vi "Bias Shift.vi"(8 "y":dbl, 9 "x":dbl, 11 "Dx, Dy":cluster{"Dx":sgl, "Dy":sgl}={"Dx"=1e-10, "Dy"=1e-10}) -> (2 "Y (m)":sgl format="%.3p", 3 "X (m)":sgl format="%.3p")   [LabVIEW 2025]
uses:
  <userlib>/Nanonis Prog Interface V5e/Nanonis Prog Interface.lvlib
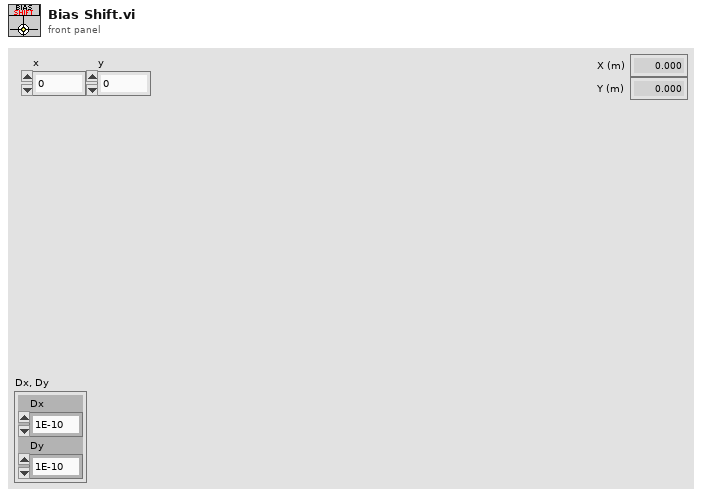
[diagram p1: front panel]
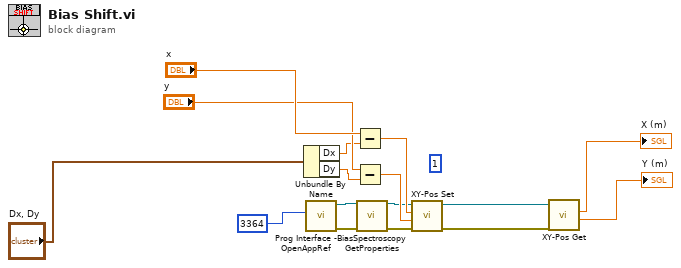
[diagram p0: block diagram]
diagram:
  (unwired) 1
  n1 = Unbundle By Name("Dx, Dy") -> ("Dx"=w2:sgl, "Dy"=w1:sgl)
  n2 = call <userlib>:"Prog Interface - OpenAppRef.vi"("Port number (3364)"=u32 3364) -> ("Error out"=w13:errorcluster, "Application reference"=w14:refnum<vi>)  [unwired: 5 in]
  n3 = Subtract(x="x", y=w2) -> (x-y=w16:dbl)
  n4 = Subtract(x="y", y=w1) -> (x-y=w15:dbl)
  n5 = call <userlib>:"BiasSpectroscopy GetProperties.vi"("Application ref in"=w14, "Error in (no error)"=w13) -> ("Application ref out"=w12:refnum<vi>, "Error out"=w11:errorcluster)  [unwired: 6 in, 6 out]
  n6 = call <userlib>:"XY-Pos Set.vi"("error in (no error)"=w11, "Y (m)"=w15, "X (m)"=w16, "Application ref in"=w12) -> ("error out"=w4:errorcluster, "Application ref out"=w5:refnum<vi>)  [unwired: 4 in]
  n7 = call <userlib>:"XY-Pos Get.vi"("error in (no error)"=w4, "Application ref in"=w5) -> ("Y (m)"=→"Y (m)":sgl, "X (m)"=→"X (m)":sgl)  [unwired: 5 in, 2 out]
